vi "execute.vi"(8 "error in (no error)":errorcluster, 9 "B in":refnum<class "GenericComponent.lvclass">, 10 "A in":refnum<class "GenericComponent.lvclass">, 11 "GenericAdapter in":refnum<class "GenericAdapter.lvclass">) -> (0 "error out":errorcluster, 1 "B out":refnum<class "GenericComponent.lvclass">, 2 "A out":refnum<class "GenericComponent.lvclass">, 3 "GenericAdapter out":refnum<class "GenericAdapter.lvclass">)   [LabVIEW 2010, in "GenericAdapter.lvclass"]
uses:
  GenericAdapter.lvclass
  common/classes/GenericComponent/GenericComponent/GenericComponent.lvclass
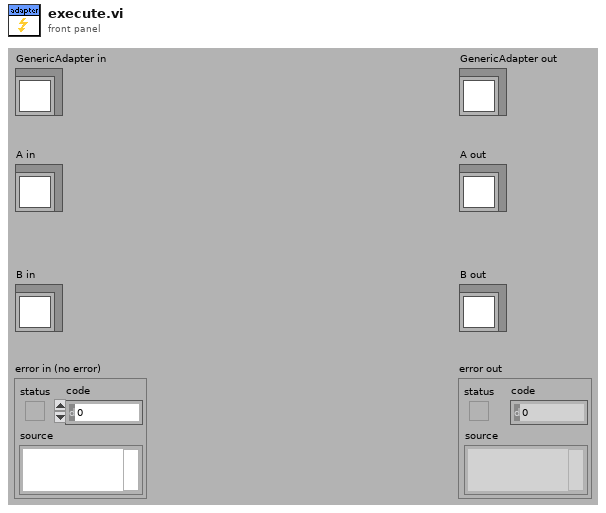
[diagram p1: front panel]
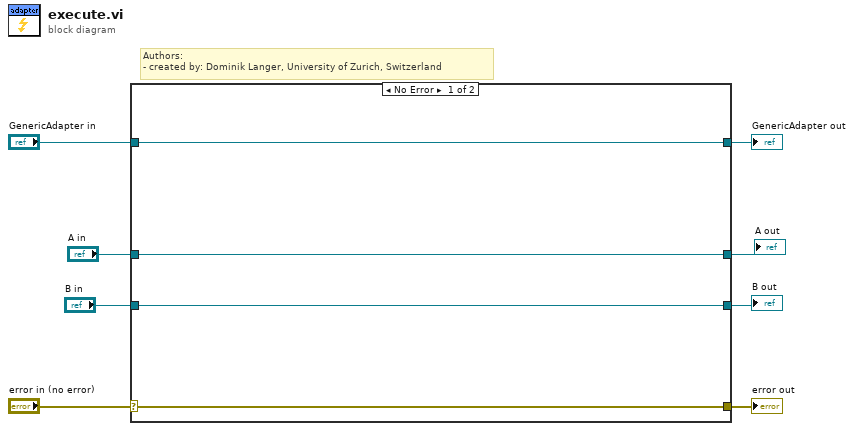
[diagram p0: block diagram]
diagram:
  # "Authors: \n- created by: Dominik Langer, University of Zurich, Switzerland"
  n1 = case shown="No Error" "error in (no error)" {
    selector: "error in (no error)" -> [w11 w16]
    tunnel: [w11 w16] -> w7
    tunnel: [w12 w15] -> w5
    tunnel: "GenericAdapter in" -> [w12 w15]
    tunnel: [w10 w13] -> w2
    tunnel: "A in" -> [w10 w13]
    tunnel: [w9 w14] -> w1
    tunnel: "B in" -> [w9 w14]
    frame No Error {
    }
    frame Error {
    }
  }
  "error out" <- w7
  "GenericAdapter out" <- w5
  "A out" <- w2
  "B out" <- w1
